vi "Configure Output.vi"(0 "VISA resource name":refnum<visa-resource-name>, 1 "Manual Range(0.00)":dbl format="%.2f", 5 "Channel Select":enum16{"Channel 1", "Channel 2", "Channel 3"}(ring), 7 "Function(0:Voltage)":u16(ring) items=["Voltage", "Current"], 9 "Enable Output (T: Enable)":bool=TRUE, 11 "error in (no error)":errorcluster, 12 "Unit(V)":u16(ring) items=["V", "mV", "kV", "A", "mA"]) -> (4 "VISA resource name out":refnum<visa-resource-name>, 15 "error out":errorcluster)   [LabVIEW 2018, in "Keithley KE22xx Series.lvlib"]
doc: "Configure voltage or current value.\nSelect the output on/off and then set the Voltage or current value as per the selection of the voltage and current."
uses:
  Keithley KE22xx Series.lvlib
panel:
  # "© 2012 Keithley Instruments, Inc. ALL RIGHTS RESERVED"
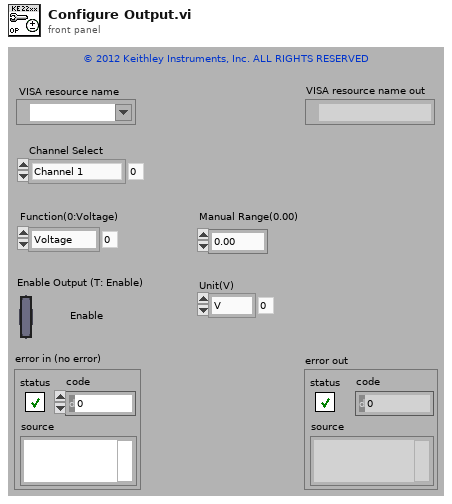
[diagram p1: front panel]
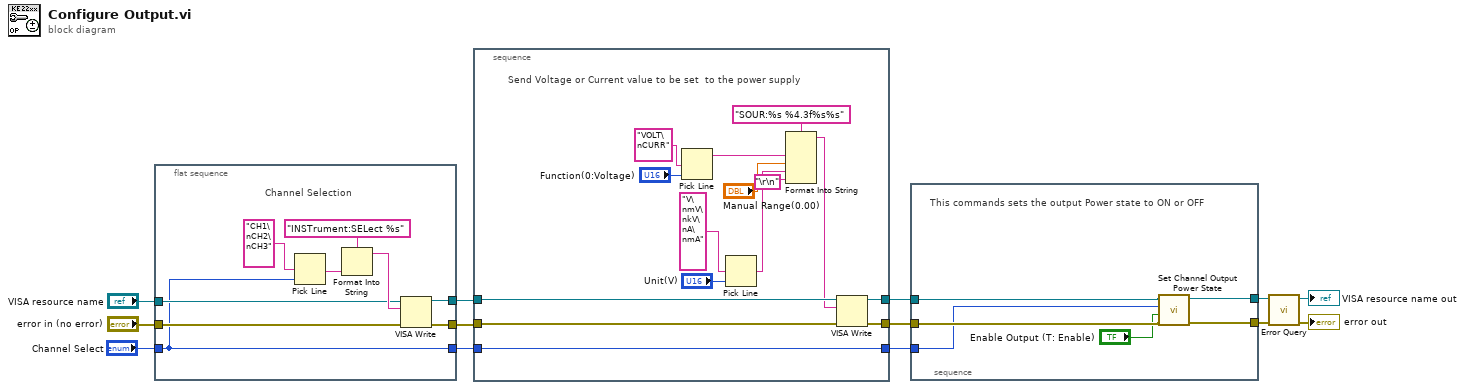
[diagram p0: block diagram]
diagram:
  n1 = flat-sequence {
    tunnel: "VISA resource name" -> [w15]
    tunnel: "error in (no error)" -> [w18]
    tunnel: [w17] -> w8
    tunnel: [w16] -> w9
    tunnel: "Channel Select" -> [w14]
    tunnel: [w14] -> w2
    frame #0 {
      # "Channel Selection"
      n2 = Pick Line(multi-line string="CH1\nCH2\nCH3", line index=w14) -> (output string=w19:string)  [unwired: 1 in]
      n3 = Format Into String(format string="INSTrument:SELect %s", w19) -> (resulting string=w21:string)  [unwired: 2 in, 1 out]
      n4 = VISA Write(VISA resource name=w15, write buffer=w21, error in (no error)=w18) -> (VISA resource name out=w16:refnum<visa-resource-name>, error out=w17:errorcluster)  [unwired: 1 out]
    }
  }
  n5 = stacked-sequence {
    tunnel: [w37] -> w7
    tunnel: [w36] -> w6
    tunnel: w9 -> [w29]
    tunnel: w8 -> [w28]
    tunnel: w2 -> [w23]
    tunnel: [w23] -> w1
    frame #0 {
      # "Send Voltage or Current value to be set  to the power supply"
      n6 = Pick Line(multi-line string="VOLT\nCURR" ("format string"), line index="Function(0:Voltage)") -> (output string=w30:string)  [unwired: 1 out]
      n7 = Pick Line(multi-line string="V\nmV\nkV\nA\nmA", line index="Unit(V)") -> (output string=w31:string)  [unwired: 1 out]
      n8 = Format Into String(format string="SOUR:%s %4.3f%s%s", w30, "Manual Range(0.00)", w31, "\r\n") -> (resulting string=w24:string)  [unwired: 2 in, 1 out]
      n9 = VISA Write(VISA resource name=w29, write buffer=w24, error in (no error)=w28) -> (VISA resource name out=w37:refnum<visa-resource-name>, error out=w36:errorcluster)  [unwired: 1 out]
    }
  }
  n10 = stacked-sequence {
    tunnel: w7 -> [w43]
    tunnel: w6 -> [w41]
    tunnel: [w42] -> w5
    tunnel: [w40] -> w4
    tunnel: w1 -> [w38]
    frame #0 {
      # "This commands sets the output Power state to ON or OFF"
      n11 = call "Set Channel Output Power State.vi"("error in (no error)"=w41, "Enable Output (T: On)"="Enable Output (T: Enable)", "Channel Select"=w38, "Visa Resource Name IN"=w43) -> ("error out"=w40:errorcluster, "Visa Resource Name OUT"=w42:refnum<visa-resource-name>)  [unwired: 6 in]
    }
  }
  n12 = call "Error Query.vi"("error in (no error)"=w4, "VISA resource name"=w5) -> ("error out"=→"error out":errorcluster, "VISA resource name out"=→"VISA resource name out":refnum<visa-resource-name>)  [unwired: 6 in, 2 out]
